vi "Picture Config Dialog.vi"(8 "error in (no error)":errorcluster, 11 "Picture Config In":T1) -> (0 "error out":errorcluster, 3 "Picture Config Out":T1)   [LabVIEW 2017]
uses:
  Picture Configuration.ctl
panel:
  in  "Scale":dbl(slide)=1.0 scale=0.01..100.0
  in  "Rotation (deg)":dbl
  in  "Rotation Y":i32
  in  "Rotation X":i32
  in  "Offset Y":i32
  in  "Offset X":i32
  in  "Cancel Button":bool
  in  "OK Button":bool
  in  "Image Path":path
  out "Image Preview":picture caption="Image Preview (Top Left)"
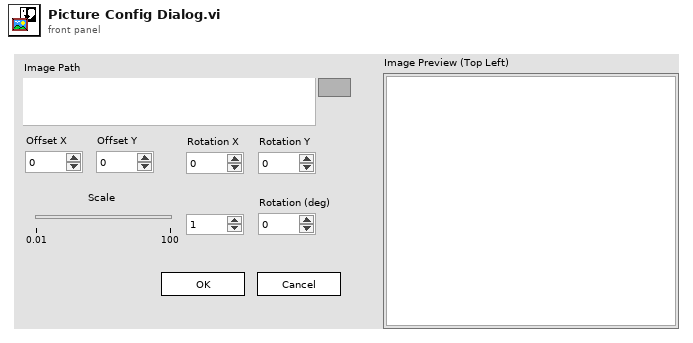
[diagram p1: front panel]
types:
  T1 = typedef "Picture Configuration.ctl" = cluster{"Path":path, "Start Pixels":cluster{"X":i32, "Y":i32}, "Rotation":dbl, "Rotation Pixels":cluster{"X":i32, "Y":i32}, "Scale":dbl}
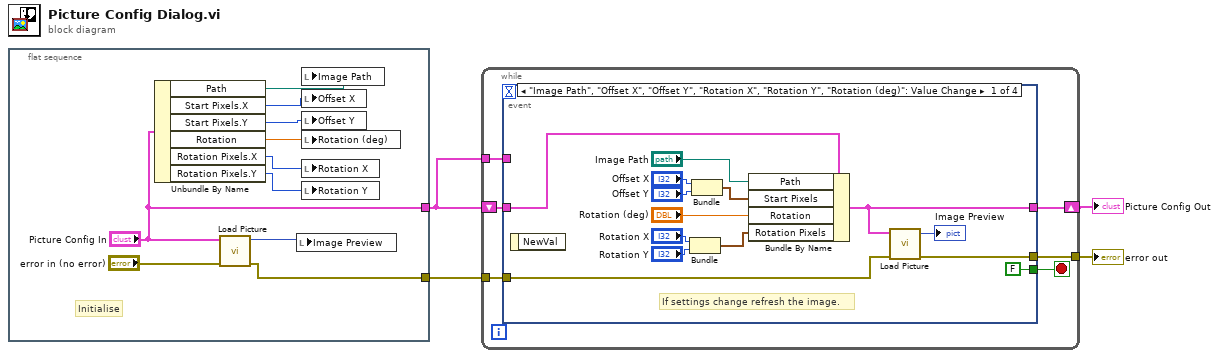
[diagram p0: block diagram]
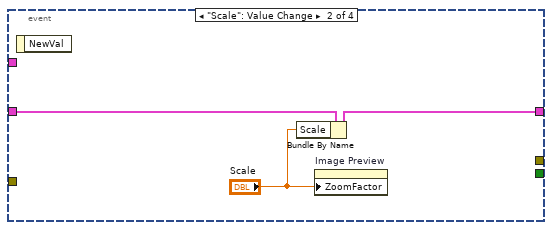
[diagram p2: hidden frame]
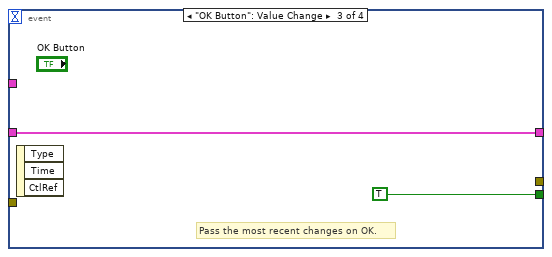
[diagram p3: hidden frame]
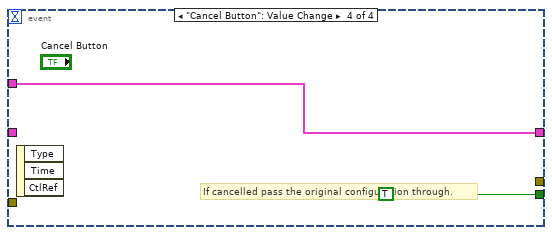
[diagram p4: hidden frame]
diagram:
  n1 = flat-sequence {
    tunnel: ["Picture Config In"] -> w3
    tunnel: [w10] -> w2
    frame #0 {
      # "Initialise"
      n2 = Unbundle By Name("Picture Config In") -> ("Path"=w12:path, "Start Pixels.X"=w9:i32, "Start Pixels.Y"=w8:i32, "Rotation"=w7:dbl, "Rotation Pixels.X"=w6:i32, "Rotation Pixels.Y"=w5:i32)
      n3 = call "Load Picture.vi"("error in (no error)"="error in (no error)", "Picture Config"="Picture Config In") -> ("error out"=w10:errorcluster, "Picture from File"=w13:picture)  [unwired: 8 in]
      n4 = local write "Image Preview"(w13) -> ()
      n5 = local write "Image Path"(w12) -> ()
      n6 = local write "Offset X"(w9) -> ()
      n7 = local write "Offset Y"(w8) -> ()
      n8 = local write "Rotation (deg)"(w7) -> ()
      n9 = local write "Rotation X"(w6) -> ()
      n10 = local write "Rotation Y"(w5) -> ()
    }
  }
  n11 = while {
    shift-right: [w19] -> w4
    shift-left: w3 -> [w18]
    tunnel: w3 -> [w20]
    tunnel: w2 -> [w16]
    tunnel: [w15] -> w1
    stop <- w17 stop-if-true
    n12 = event shown="[0] \"Image Path\", \"Offset X\", \"Offset Y\", \"Rotation X\", \"Rotation Y\", \"Rotation (deg)\": Value Change" {
      selector: _ -> [_ _ _ _]
      dyn-events: _ -> [_ _ _ _]
      timeout: _ -> [_ _ _ _]
      tunnel: w20 -> [_ _ _ w41]
      tunnel: [w32 w35 w39 w41] -> w19
      tunnel: w18 -> [w25 w37 w39 _]
      tunnel: [FALSE _ TRUE TRUE] -> w17
      tunnel: w16 -> [w31 _ _ _]
      tunnel: [w30 _ _ _] -> w15
      event "Image Path", "Offset X", "Offset Y", "Rotation X", "Rotation Y", "Rotation (deg)": Value Change {
        # "If settings change refresh the image."
        n13 = event-data() -> ()  [unwired: 1 in, 1 out]
        n14 = Bundle("Rotation X"="Rotation X", "Rotation Y"="Rotation Y") -> (w21:cluster{"Rotation X":i32, "Rotation Y":i32})  [unwired: 1 in]
        n15 = Bundle("Offset X"="Offset X", "Offset Y"="Offset Y") -> (w26:cluster{"Offset X":i32, "Offset Y":i32})  [unwired: 1 in]
        n16 = Bundle By Name(cluster=w25, "Path"="Image Path", "Start Pixels"=w26, "Rotation"="Rotation (deg)", "Rotation Pixels"=w21) -> (w32:T1)
        n17 = call "Load Picture.vi"("error in (no error)"=w31, "Picture Config"=w32) -> ("error out"=w30:errorcluster, "Picture from File"=→"Image Preview":picture)  [unwired: 8 in]
      }
      event "Scale": Value Change {
        n18 = event-data() -> ()  [unwired: 1 in, 1 out]
        n19 = Bundle By Name(cluster=w37, "Scale"="Scale") -> (w35:T1)
        n20 = property on="Image Preview" class="Pict"("ZoomFactor"="Scale") -> ()  [unwired: 2 in, 2 out]
      }
      event "OK Button": Value Change {
        # "Pass the most recent changes on OK."
        n21 = event-data() -> ()  [unwired: 1 in, 3 out]
      }
      event "Cancel Button": Value Change {
        # "If cancelled pass the original configuration through."
        n22 = event-data() -> ()  [unwired: 1 in, 3 out]
      }
    }
  }
  "Picture Config Out" <- w4
  "error out" <- w1
